vi "Get Error Shifter from While Loop.vi"(8 "error in (no error)":errorcluster, 11 "WhileLoop":refnum<vi>) -> (0 "error out":errorcluster, 2 "Error Cluster Shift Register":refnum<vi>)   [LabVIEW 2020, in "JKI State Machine API.lvlib" / "JKI SM.lvclass"]
uses:
  JKI SM/JKI SM.lvclass
  JKI SM/JKI SM.lvclass/JKI SM.ctl
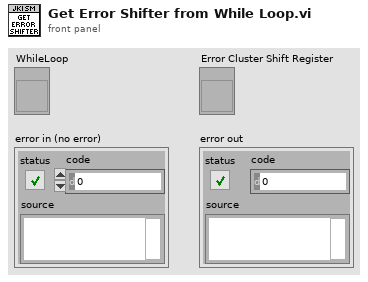
[diagram p1: front panel]
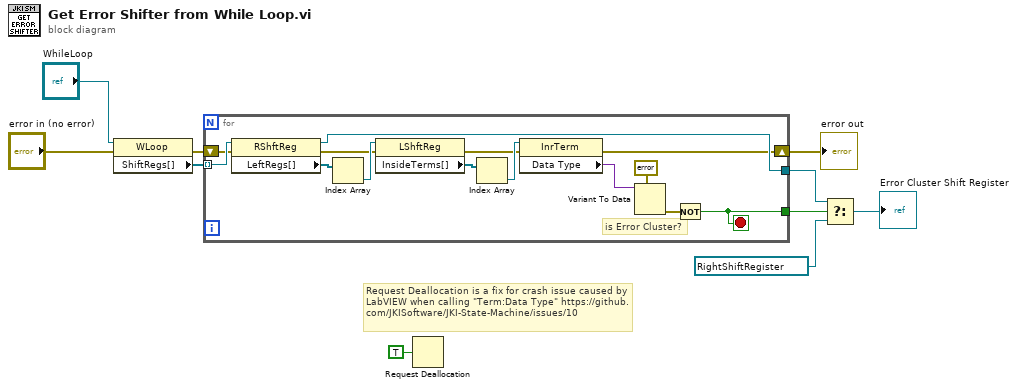
[diagram p0: block diagram]
diagram:
  # "Request Deallocation is a fix for crash issue caused by LabVIEW when calling \"Term:Data Type\" https://github.com/JKISoftware/JKI-State-Machine/issues/10"
  n1 = property class="WLoop"(reference="WhileLoop", error in="error in (no error)") -> (error out=w6:errorcluster, "ShiftRegs[]"=w2:refnum<vi>[])  [unwired: 1 out]
  n2 = for {
    tunnel: w2 -> [w24] mode=indexing
    tunnel: [w16] -> w4
    tunnel: [w15] -> w3
    shift-right: [w11] -> w8
    shift-left: w6 -> [w14]
    stop <- w15 stop-if-true
    # "is Error Cluster?"
    n3 = property class="RShftReg"(reference=w24, error in=w14) -> (reference out=w16:refnum<vi>, error out=w13:errorcluster, "LeftRegs[]"=w23:refnum<vi>[])
    n4 = Index Array(array=w23) -> (element=w22:refnum<vi>)  [unwired: 1 in]
    n5 = property class="LShftReg"(reference=w22, error in=w13) -> (error out=w12:errorcluster, "InsideTerms[]"=w21:refnum<vi>[])  [unwired: 1 out]
    n6 = Index Array(array=w21) -> (element=w20:refnum<vi>)  [unwired: 1 in]
    n7 = property class="InrTerm"(reference=w20, error in=w12) -> (error out=w11:errorcluster, "Data Type"=w18:variant)  [unwired: 1 out]
    n8 = Variant To Data(type=errorcluster {"status"=FALSE, "code"=0, "source"=""} ("error in (no error)"), Variant=w18) -> (error out=w17:errorcluster)  [unwired: 1 in, 1 out]
    n9 = Not(x=w17) -> (.not. x?=w15:bool)
  }
  "error out" <- w8
  n10 = Request Deallocation(TRUE ("flag")) -> ()
  n11 = Select(t=w4, s=w3, f=refnum<vi> refnum) -> (s? t:f=→"Error Cluster Shift Register":refnum<vi>)
